vi "Calibration-Frame15.vi"(9 "Array 8":dbl[](array[numeric]), 10 "data mode":enum16{"Take new data point", "Refit Curve"}(ring), 11 "Results file output":path) -> ()   [LabVIEW 2015]
uses:
  Anemometry Sub Vis/Controls/App_Global.ctl
  Anemometry Sub Vis/Controls/Setup.ctl
  Anemometry Sub Vis/Controls/Post_Process.ctl
  Anemometry Sub Vis/Controls/Save_Data.ctl
  Anemometry Sub Vis/File/Setup_Filetype.ctl
  Anemometry Sub Vis/Globals/Calib_global.vi
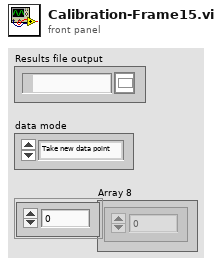
[diagram p1: front panel]
types:
  T1 = typedef "App_Global.ctl" = enum16{"Read Global", "Write to Global", "Initialise Array"}
  T2 = typedef "Save_Data.ctl" = enum16{"Save No Data", "Save Data"}
  T3 = typedef "Post_Process.ctl" = enum16{"Take New Data", "Post Process Raw Data File"}
  T4 = typedef "Setup.ctl" = enum16{"Run Program", "Show Setup", "Save Current Setup", "Setup Front Panel"}
  T5 = typedef "Setup_Filetype.ctl" = enum16{"Measurement Setups", "Calibration Setups", "General", "Results File Plotter Setups", "Speed Calib Tweaks"}
  T6 = typedef "Cal_Inst_type.ctl" = enum16{"Propeller anemometer", "Pressure Transducer", "Hot wire", "Cross wire velocity", "Cross wire angle", "Generic Linear", "Generic Polynomial", "Generic BackPoly", "Fast FID", "Thermocouple", "Cold wire", "Pulsed Wire"}
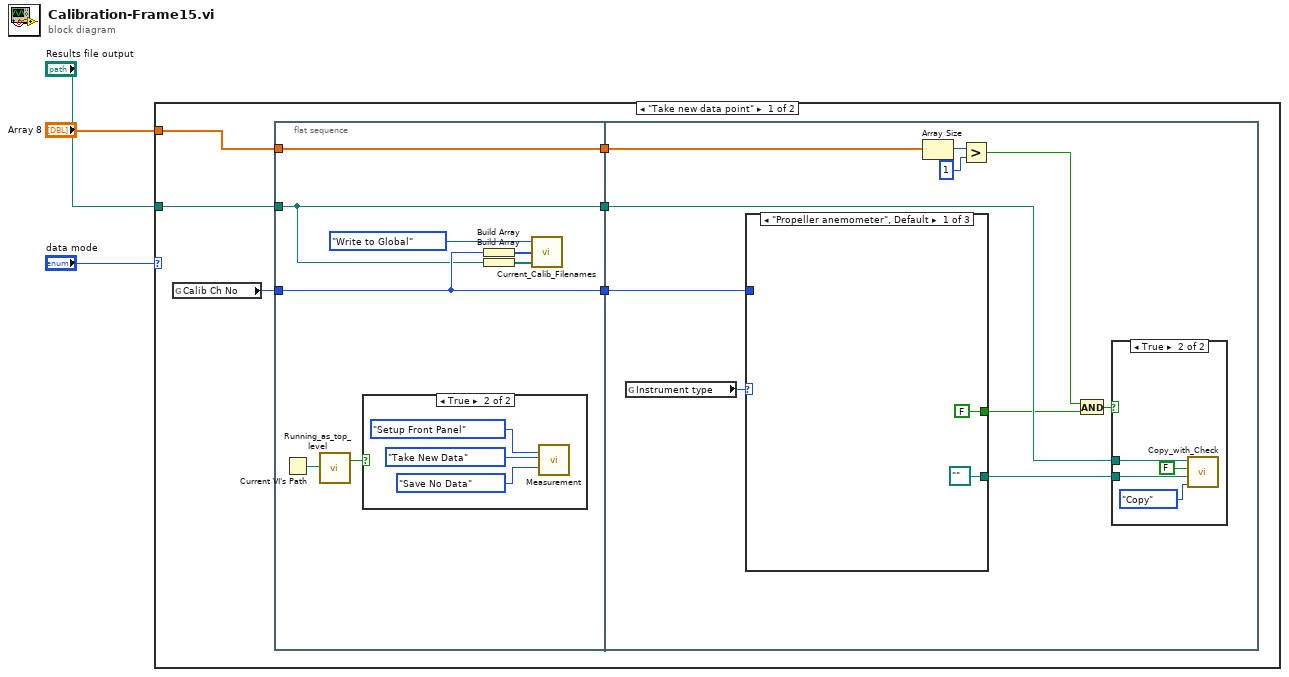
[diagram p0: block diagram]
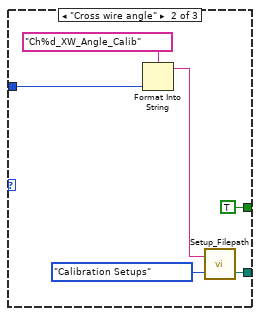
[diagram p4: hidden frame]
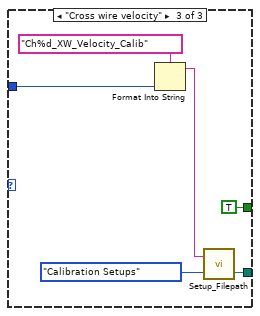
[diagram p5: hidden frame]
diagram:
  n1 = case shown="\"Take new data point\"" "data mode" {
    tunnel: "Results file output" -> [w9 _]
    tunnel: "Array 8" -> [w5 _]
    frame "Take new data point" {
      n2 = global read "Calib_global.vi" "Calib Ch No"() -> (w8:i16)
      n3 = flat-sequence {
        tunnel: w9 -> [w11]
        tunnel: [w11] -> w7
        tunnel: w8 -> [w12]
        tunnel: [w12] -> w6
        tunnel: w5 -> [w10]
        tunnel: [w10] -> w4
        tunnel: w7 -> [w28]
        tunnel: w6 -> [w22]
        tunnel: w4 -> [w21]
        frame #0 {
          n4 = Current VI's Path() -> (path=w17:path)
          n5 = call "Running_as_top_level.vi"("Vi path name"=w17) -> ("Top Level"=w16:bool)  [unwired: 1 out]
          n6 = case shown="True" w16 {
            frame False {
            }
            frame True {
              n7 = call "Measurement.vi"("setup"=Setup."Setup Front Panel", "Post Process"=Post_Process."Take New Data", "File"=Save_Data."Save No Data") -> ()  [unwired: 4 in, 13 out]
            }
          }
          n8 = Build Array(w12) -> (w14:i16[])
          n9 = Build Array(w11) -> (w15:path[])
          n10 = call "Current_Calib_Filenames.vi"("Calib Filename"=w15, "Channel Numbers"=w14, "Mode"=App_Global."Write to Global") -> ()  [unwired: 3 out]
        }
        frame #1 {
          n11 = global read "Calib_global.vi" "Instrument type"() -> (w30:T6)
          n12 = case shown="\"Propeller anemometer\", Default" w30 {
            tunnel: w22 -> [_ w42 w48]
            tunnel: [path "" ("appended path") w38 w43] -> w29
            tunnel: [FALSE TRUE TRUE] -> w25
            frame "Propeller anemometer", Default {
            }
            frame "Cross wire angle" {
              n13 = Format Into String(format string="Ch%d_XW_Angle_Calib", w42) -> (resulting string=w37:string)  [unwired: 2 in, 1 out]
              n14 = call "Setup_Filepath.vi"("Setup File Type"=Setup_Filetype."Calibration Setups", "Filename in"=w37) -> ("Filename Out"=w38:path)  [unwired: 1 out]
            }
            frame "Cross wire velocity" {
              n15 = Format Into String(format string="Ch%d_XW_Velocity_Calib", w48) -> (resulting string=w44:string)  [unwired: 2 in, 1 out]
              n16 = call "Setup_Filepath.vi"("Setup File Type"=Setup_Filetype."Calibration Setups", "Filename in"=w44) -> ("Filename Out"=w43:path)  [unwired: 1 out]
            }
          }
          n17 = Array Size(array=w21) -> (size(s)=w27:i32)
          n18 = Greater?(x=w27, y=1) -> (0:w24:bool)
          n19 = And(x=w24, y=w25) -> (x .and. y?=w23:bool)
          n20 = case shown="True" w23 {
            tunnel: w29 -> [_ w33]
            tunnel: w28 -> [_ w32]
            frame False {
            }
            frame True {
              n21 = call "Copy_with_Check.vi"("Mode"=enum16{"Move", "Copy"}."Copy", "Target Path"=w33, "Variable Target?"=FALSE, "Source Path"=w32) -> ()  [unwired: 1 out]
            }
          }
        }
      }
    }
    frame "Refit Curve" {
    }
  }
